vi "camera_change_ROI.vi"(6 "BufferInterval":u32, 8 "error in":errorcluster, 9 "Region of Interest":i32[](array[numeric]), 10 "Ereignisregistrierung (Referenz) 2":refnum<event-registration>, 11 "Session In":T1) -> (0 "Fehler (Ausgang)":errorcluster, 2 "Ereignisregistrierung (Referenz)":refnum<event-registration>, 3 "Session Out":T1)   [LabVIEW 2009]
uses:
  <vilib>/userDefined/High Color/IMAQdx.ctl
  C:/Program Files/National Instruments/LabVIEW 2009/resource/objmgr/imaqdx.rc
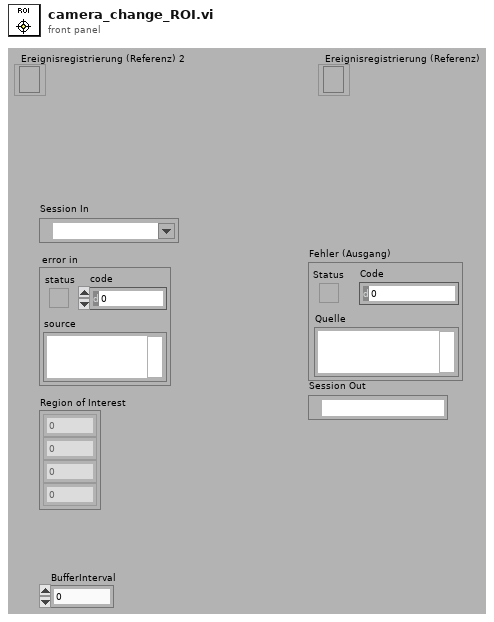
[diagram p1: front panel]
types:
  T1 = typedef "IMAQdx.ctl" = refnum<k21>
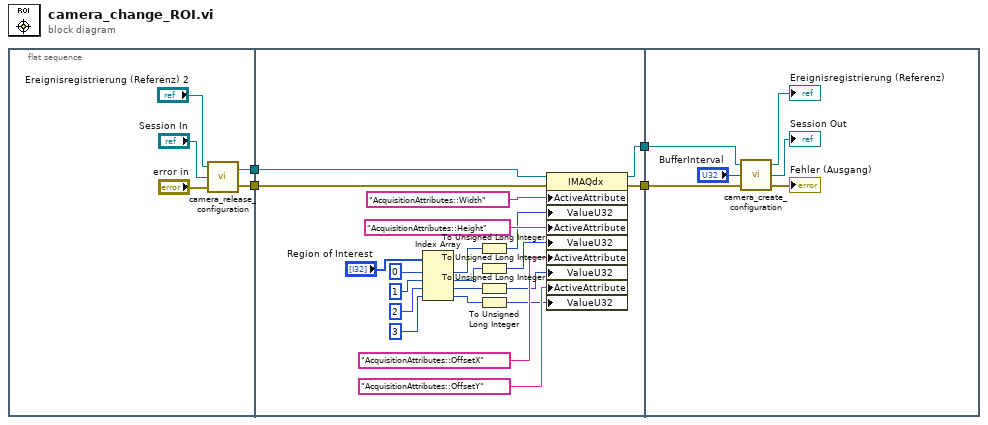
[diagram p0: block diagram]
diagram:
  n1 = flat-sequence {
    tunnel: [w9] -> w4
    tunnel: [w8] -> w3
    tunnel: w4 -> [w14]
    tunnel: w3 -> [w13]
    tunnel: [w12] -> w2
    tunnel: [w10] -> w1
    tunnel: w2 -> [w36]
    tunnel: w1 -> [w34]
    frame #0 {
      n2 = call "camera_release_configuration.vi"("error in"="error in", "Session In"="Session In", "Ereignisregistrierung (Referenz) 2"="Ereignisregistrierung (Referenz) 2") -> ("error out"=w9:errorcluster, "Session Out"=w8:T1)
    }
    frame #1 {
      n3 = Index Array(array="Region of Interest", index #1=0 ("Index"), index #2=1 ("Index"), index #3=2 ("Index"), index #4=3 ("Index")) -> (element #1=w20:i32, element #2=w21:i32, element #3=w17:i32, element #4=w22:i32)
      n4 = To Unsigned Long Integer(number=w20) -> (unsigned 32bit integer=w19:u32)
      n5 = To Unsigned Long Integer(number=w21) -> (unsigned 32bit integer=w18:u32)
      n6 = To Unsigned Long Integer(number=w17) -> (unsigned 32bit integer=w16:u32)
      n7 = To Unsigned Long Integer(number=w22) -> (unsigned 32bit integer=w15:u32)
      n8 = property class="IMAQdx"(reference=w13, error in=w14, "ActiveAttribute"="AcquisitionAttributes::Width", "ValueU32"=w19, "ActiveAttribute"="AcquisitionAttributes::Height", "ValueU32"=w18, "ActiveAttribute"="AcquisitionAttributes::OffsetX", "ValueU32"=w16, "ActiveAttribute"="AcquisitionAttributes::OffsetY", "ValueU32"=w15) -> (reference out=w12:T1, error out=w10:errorcluster)
    }
    frame #2 {
      n9 = call "camera_create_configuration.vi"("error in"=w34, "BufferInterval"="BufferInterval", "Session Out 2"=w36) -> ("Fehler (Ausgang)"=→"Fehler (Ausgang)":errorcluster, "Session Out"=→"Session Out":T1, "Ereignisregistrierung (Referenz)"=→"Ereignisregistrierung (Referenz)":refnum<event-registration>)
    }
  }
